vi "Destroy Generic Optimization User Events.vi"(8 "error in":errorcluster, 11 "Generic Optimization in":refnum<class "Generic Optimization.lvclass">) -> (0 "error out":errorcluster, 3 "Generic Optimization out":refnum<class "Generic Optimization.lvclass">)   [LabVIEW 2016]
uses:
  Generic Optimization.lvclass
  C:/Users/Administrator/Desktop/LabVIEW EMS/SCADA Sub Abstract Actor/SCADA Sub Abstract/SCADA Sub Abstract.lvclass
  C:/Users/Administrator/Desktop/LabVIEW EMS/EMS Generic Actor/EMS Generic/EMS Generic.lvclass
  C:/Program Files (x86)/National Instruments/LabVIEW 2016/vi.lib/ActorFramework/Actor/Actor.lvclass
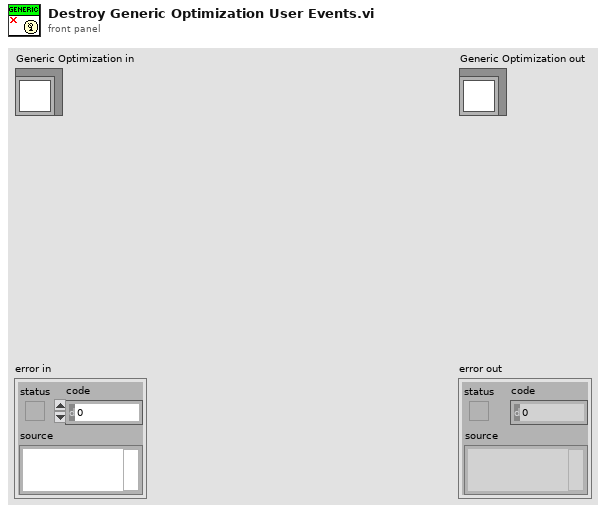
[diagram p1: front panel]
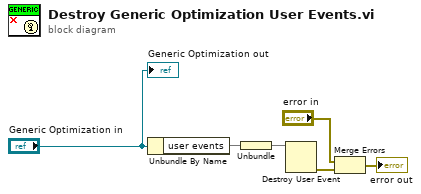
[diagram p0: block diagram]
diagram:
  n1 = Unbundle By Name("Generic Optimization in") -> ("user events"=w5)
  n2 = Unbundle(w5) -> (w4)
  n3 = Destroy User Event(user event=w4) -> (error out=w2:errorcluster)  [unwired: 1 in]
  n4 = Merge Errors("error in", w2) -> (→"error out":errorcluster)
  "Generic Optimization out" <- "Generic Optimization in"
